vi "MessageName.vi"() -> (2 "MessageName":string)   [LabVIEW 2020, in "Service.lvlib"]
uses:
  Service.lvlib
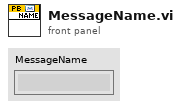
[diagram p1: front panel]
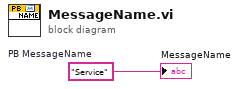
[diagram p0: block diagram]
diagram:
  w1 = "Service"  # PB MessageName
  "MessageName" <- w1
